vi "VI Bookmarks.vi"(8 "Error In":errorcluster, 10 "VIs":T2[](array[typedef]), 11 "Project Target App In":refnum<vi>) -> (0 "Error Out":errorcluster, 2 "VI Bookmarks":T1[](array[typedef]), 3 "Project Target App Out":refnum<vi>)   [LabVIEW 2017, in "Bookmark Manager.lvlib"]
uses:
  Bookmark Manager.lvlib
  VI Information.ctl
  Application Information.ctl
  VI Bookmark.ctl
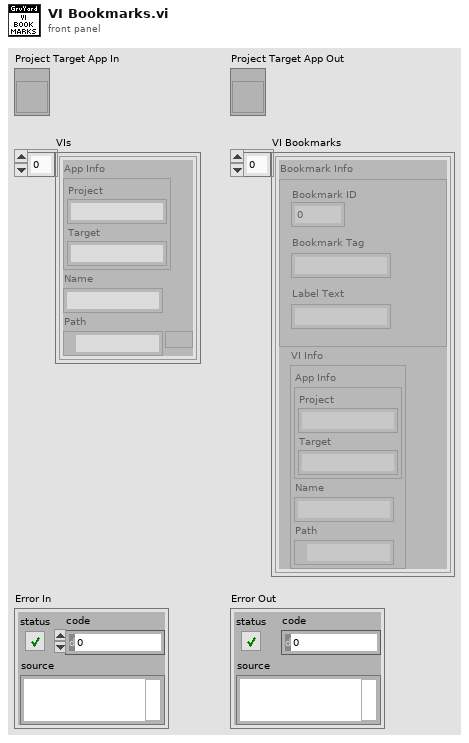
[diagram p1: front panel]
types:
  T1 = typedef "Bookmark Manager.lvlib/VI Bookmark.ctl" = cluster{"Bookmark Info":cluster{"Bookmark ID":u32, "Bookmark Tag":string, "Label Text":string}, "VI Info":T2}
  T2 = typedef "Bookmark Manager.lvlib/VI Information.ctl" = cluster{"App Info":T3, "Name":string, "Path":path}
  T3 = typedef "Bookmark Manager.lvlib/Application Information.ctl" = cluster{"Project":string, "Target":string}
  T4 = typedef "LVBookmarkInfoTypeDef.ctl" = cluster{"Bookmark Reference":u32, "Bookmark Tag":string, "Label Text":string}[]
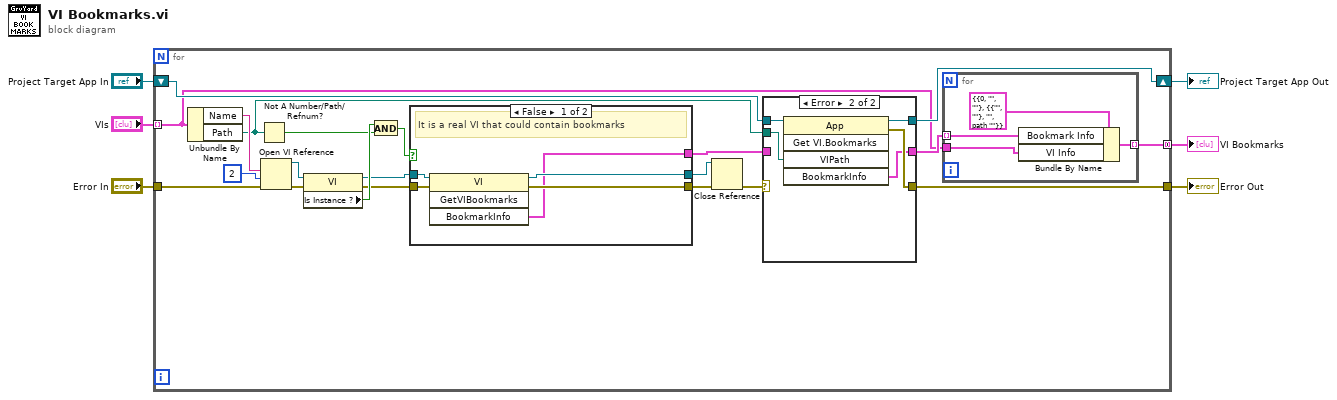
[diagram p0: block diagram]
diagram:
  n1 = for {
    tunnel: "Error In" -> [w27]
    tunnel: "VIs" -> [w10] mode=indexing
    shift-right: [w12] -> w6
    shift-left: "Project Target App In" -> [w13]
    tunnel: [w9] -> w5
    tunnel: [w8] -> w1 mode=concatenating
    n2 = Unbundle By Name(w10) -> ("Name"=w15:string, "Path"=w14:path)
    n3 = Not A Number/Path/Refnum?(number/path/refnum=w14) -> (NaN/Path/Refnum?=w22:bool)
    n4 = Open VI Reference(vi path=w15, options=2, error in (no error)=w27) -> (vi reference=w24:refnum<vi>, error out=w25:errorcluster)  [unwired: 3 in]
    n5 = property class="VI"(reference=w24, error in=w25) -> (reference out=w19:refnum<vi>, error out=w20:errorcluster, "Is Instance ?"=w23:bool)
    n6 = And(x=w23, y=w22) -> (x .and. y?=w21:bool)
    n7 = case shown="False" w21 {
      tunnel: w20 -> [w43 w45]
      tunnel: w19 -> [w44 w46]
      tunnel: [w42 w46] -> w7
      tunnel: [w41 w45] -> w18
      tunnel: [w40 _] -> w16
      frame False {
        # "It is a real VI that could contain bookmarks"
        n8 = invoke class="VI" method="GetVIBookmarks"(reference=w44, error in=w43) -> (reference out=w42:refnum<vi>, error out=w41:errorcluster, "BookmarkInfo"=w40:T4)  [unwired: 2 in, 1 out]
      }
      frame True {
        # "It is an Express VI or the path does not exist"
      }
    }
    n9 = Close Reference(reference=w7, error in (no error)=w18) -> (error out=w17:errorcluster)
    n10 = case shown="Error" w17 {
      selector: w17 -> [w33 _]
      tunnel: w16 -> [w34 _]
      tunnel: [w34 w38] -> w11
      tunnel: [w33 w39] -> w9
      tunnel: w14 -> [_ w37]
      tunnel: w13 -> [w32 w36]
      tunnel: [w32 w35] -> w12
      frame No Error {
      }
      frame Error {
        n11 = invoke class="App" method="Get VI.Bookmarks"(reference=w36, "VIPath"=w37) -> (reference out=w35:refnum<vi>, error out=w39:errorcluster, "BookmarkInfo"=w38:T4)  [unwired: 3 in, 2 out]
      }
    }
    n12 = for {
      tunnel: w11 -> [w30] mode=indexing
      tunnel: w10 -> [w29]
      tunnel: [w28] -> w8 mode=indexing
      n13 = Bundle By Name(cluster=T1 {"Bookmark Info"={"Bookmark ID"=0, "Bookmark Tag"="", "Label Text"=""}, "VI Info"={"App Info"={"Project"="", "Target"=""}, "Name"="", "Path"=path ""}} ("VI Bookmark"), "Bookmark Info"=w30, "VI Info"=w29) -> (w28:T1)
    }
  }
  "Project Target App Out" <- w6
  "Error Out" <- w5
  "VI Bookmarks" <- w1
